vi "Put Object from File.vi"(6 "Chunk size (kB)":i32=5120 min=5120, 7 "Object Parameters":T1={"Content Type"="binary/octet-stream", "ACL"=enum."private", "Storage Class"=enum."STANDARD", "User-Defined Metadata"=[]}, 8 "error in (no error)":errorcluster, 9 "File":path, 10 "Object Path":string, 11 "Bucket in":refnum<class "Bucket.lvclass">) -> (0 "error out":errorcluster, 1 "ETag":string, 2 "Location":string, 3 "Bucket out":refnum<class "Bucket.lvclass">, 4 "Version ID":string)   [LabVIEW 2015, in "NI_AWS_S3.lvlib" / "Bucket.lvclass"]
doc: "This operation <B>uploads an object from a file</B> to a bucket <B>in multiple parts</B>. You can <B>set Chunk size (kB) to limit memory usage</B> of the operation."
uses:
  Bucket.lvclass
  PUT Object Request Parameters.ctl
  ACL.ctl
  Storage Class.ctl
  Core/HTTP Request/Name Value Pair.ctl
  Multipart Upload/Multipart Upload.lvclass
  NI_AWS_S3.lvlib
  Core/HTTP Request/HTTP Request.lvclass
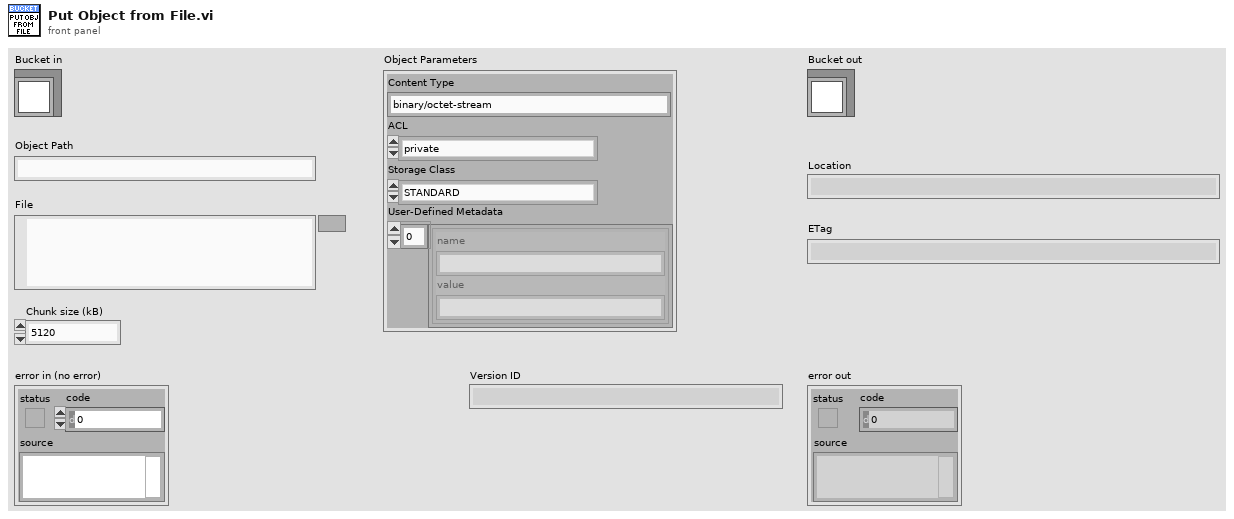
[diagram p1: front panel]
types:
  T1 = typedef "NI_AWS_S3.lvlib/PUT Object Request Parameters.ctl" = cluster{"Content Type":string, "ACL":T2, "Storage Class":T3, "User-Defined Metadata":T4[]}
  T2 = typedef "NI_AWS_S3.lvlib/ACL.ctl" = enum16{"private", "public-read", "public-read-write", "aws-exec-read", "authenticated-read", "bucket-owner-read", "bucket-owner-full-control"}
  T3 = typedef "NI_AWS_S3.lvlib/Storage Class.ctl" = enum16{"STANDARD", "REDUCED_REDUNDANCY"}
  T4 = typedef "NI_AWS_Core.lvlib/HTTP Request.lvclass/Name Value Pair.ctl" = cluster{"name":string, "value":string}
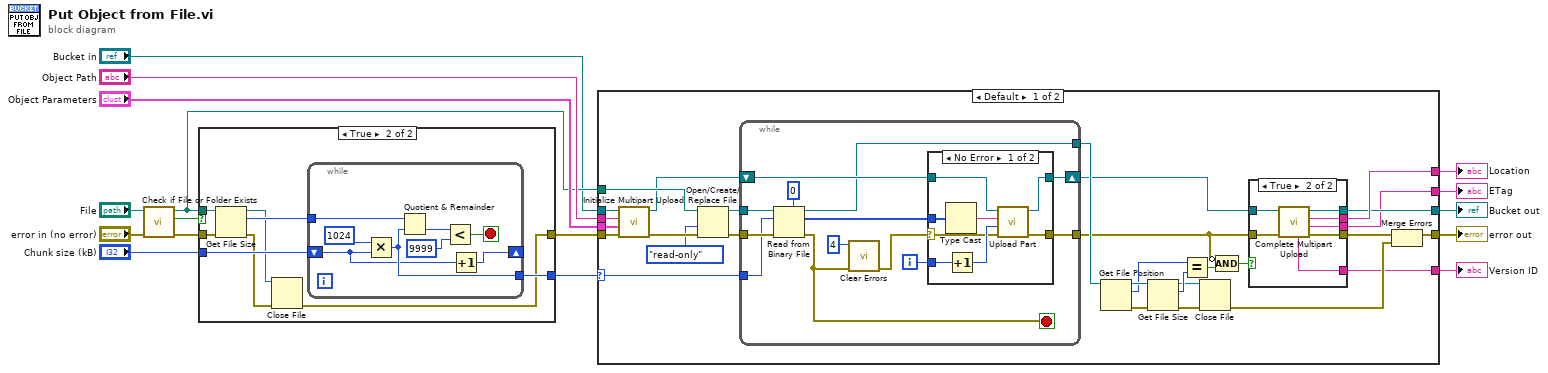
[diagram p0: block diagram]
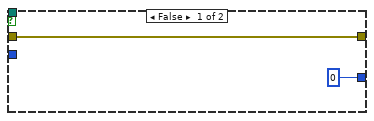
[diagram p2: hidden frame]
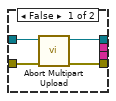
[diagram p4: hidden frame]
diagram:
  n1 = call <vilib>:"Check if File or Folder Exists.vi"("error in (no error)"="error in (no error)", "path"="File") -> ("error out"=w13:errorcluster, "file or folder exists?"=w14:bool, "dup path"=w7:path)  [unwired: 7 in]
  n2 = case shown="True" w14 {
    tunnel: w13 -> [w17 w25]
    tunnel: w7 -> [_ w26]
    tunnel: "Chunk size (kB)" -> [_ w24]
    tunnel: [0 w22] -> w11
    tunnel: [w17 w20] -> w10
    frame False {
    }
    frame True {
      n3 = Get File Size(file=w26, error in=w25) -> (refnum out=w19:refnum<file>, size (in bytes)=w23:i64, 0:w21:errorcluster)
      n4 = Close File(refnum=w19, error in=w21) -> (error out=w20:errorcluster)  [unwired: 1 out]
      n5 = while {
        tunnel: w23 -> [w34]
        shift-right: [w28] -> _
        shift-left: w24 -> [w27]
        tunnel: [w29] -> w22
        stop <- w31 stop-if-true
        n6 = Multiply(x=1024 ("y"), y=w27) -> (x*y=w29:i32)
        n7 = Quotient & Remainder(x=w34, y=w29) -> (floor(x/y)=w33:i64)  [unwired: 1 out]
        n8 = Less?(x=w33, y=i64 9999) -> (x < y?=w31:bool)
        n9 = Increment(x=w27) -> (x+1=w28:i32)
      }
    }
  }
  n10 = case shown="Default" w11 {
    selector: w11 -> [w40 _]
    tunnel: w10 -> [w63 w99]
    tunnel: "Object Path" -> [w39 _]
    tunnel: "Object Parameters" -> [w37 _]
    tunnel: w7 -> [w61 _]
    tunnel: [w42 w99] -> w6
    tunnel: [w44 _] -> w1
    tunnel: [w41 _] -> w5
    tunnel: "Bucket in" -> [w38 w98]
    tunnel: [w36 w98] -> w3
    tunnel: [w35 _] -> w2
    frame Default {
      n11 = call "Initialize Multipart Upload.vi"("error in (no error)"=w63, "PUT Object Request Parameters"=w37, "Object Path"=w39, "Bucket"=w38) -> ("error out"=w62:errorcluster, "Multipart Upload"=w60:refnum<class "Multipart Upload.lvclass">)  [unwired: 6 in]
      n12 = Open/Create/Replace File(file path (use dialog)=w61, error in=w62, access (0:read/write)=enum16{"read/write", "read-only", "write-only"}."read-only") -> (refnum out=w57:refnum<file>, error out=w58:errorcluster)  [unwired: 3 in, 1 out]
      n13 = while {
        tunnel: w58 -> [w76]
        tunnel: w57 -> [w75]
        tunnel: [w67] -> w46
        tunnel: [w66] -> w52
        tunnel: w40 -> [w69]
        shift-right: [w73] -> w48
        shift-left: w60 -> [w74]
        i -> [w72]
        stop <- w68 stop-if-true
        n14 = Read from Binary File(5:u8 0, 8:w76, 10:w69, 11:w75) -> (0:w68:errorcluster, 2:w70:u8[], 3:w66:refnum<file>)  [unwired: 2 in, 1 out]
        n15 = call <vilib>:"Clear Errors.vi"("error in (no error)"=w68, "specific error code to clear (0: all)"=4) -> ("error out"=w64:errorcluster)  [unwired: 4 in, 1 out]
        n16 = case shown="No Error" w64 {
          selector: w64 -> [w77 w85]
          tunnel: w74 -> [w84 w86]
          tunnel: [w83 w86] -> w73
          tunnel: w72 -> [w82 _]
          tunnel: w70 -> [w80 _]
          tunnel: [w78 w85] -> w67
          frame No Error {
            n17 = Type Cast(x=w80) -> (*(type *) &x=w79:string)  [unwired: 1 in]
            n18 = Increment(x=w82) -> (x+1=w81:i32)
            n19 = call "Upload Part.vi"("error in (no error)"=w77, "Part Number"=w81, "Data"=w79, "Multipart Upload in"=w84) -> ("error out"=w78:errorcluster, "Multipart Upload out"=w83:refnum<class "Multipart Upload.lvclass">)  [unwired: 6 in]
          }
          frame Error {
          }
        }
      }
      n20 = Get File Position(7:w52) -> (0:w55:errorcluster, 2:w53:i64, 3:w56:refnum<file>)  [unwired: 1 in]
      n21 = Get File Size(file=w56, error in=w55) -> (refnum out=w50:refnum<file>, size (in bytes)=w54:i64, 0:w51:errorcluster)
      n22 = Equal?(x=w53, y=w54) -> (x = y?=w49:bool)
      n23 = Close File(refnum=w50, error in=w51) -> (error out=w43:errorcluster)  [unwired: 1 out]
      n24 = Compound Arithmetic op=AND(invert w46, w49) -> (w47:bool)
      n25 = case shown="True" w47 {
        tunnel: w48 -> [w89 w96]
        tunnel: w46 -> [w90 w97]
        tunnel: [w88 w95] -> w45
        tunnel: [_ w94] -> w44
        tunnel: [_ w93] -> w41
        tunnel: [w87 w92] -> w36
        tunnel: [_ w91] -> w35
        frame False {
          n26 = call "Abort Multipart Upload.vi"("error in (no error)"=w90, "Multipart Upload"=w89) -> ("error out"=w88:errorcluster, "Bucket"=w87:refnum<class "Bucket.lvclass">)  [unwired: 8 in]
        }
        frame True {
          n27 = call "Complete Multipart Upload.vi"("error in (no error)"=w97, "Multipart Upload"=w96) -> ("error out"=w95:errorcluster, "ETag"=w91:string, "Location"=w94:string, "Bucket"=w92:refnum<class "Bucket.lvclass">, "Version ID"=w93:string)  [unwired: 5 in]
        }
      }
      n28 = Merge Errors(w45, w43) -> (w42:errorcluster)
    }
    frame 0 {
    }
  }
  "error out" <- w6
  "Version ID" <- w5
  "Bucket out" <- w3
  "ETag" <- w2
  "Location" <- w1
